vi "Delete Scale.vi"(8 "error in (no error)":errorcluster, 10 "index":i32, 11 "Polynomial Scale configuration in":refnum<class "Polynomial Scale configuration.lvclass">) -> (0 "error out":errorcluster, 3 "Polynomial Scale configuration out":refnum<class "Polynomial Scale configuration.lvclass">)   [LabVIEW 2013, in "Polynomial Scale configuration.lvclass"]
uses:
  Polynomial Scale configuration.lvclass
  <vilib>/NI/DCAF Modules/DCAF Scaling/module/configuration/Scaling configuration.lvclass
  Polynomial Scale configuration.lvclass/Polynomial Scale configuration.ctl
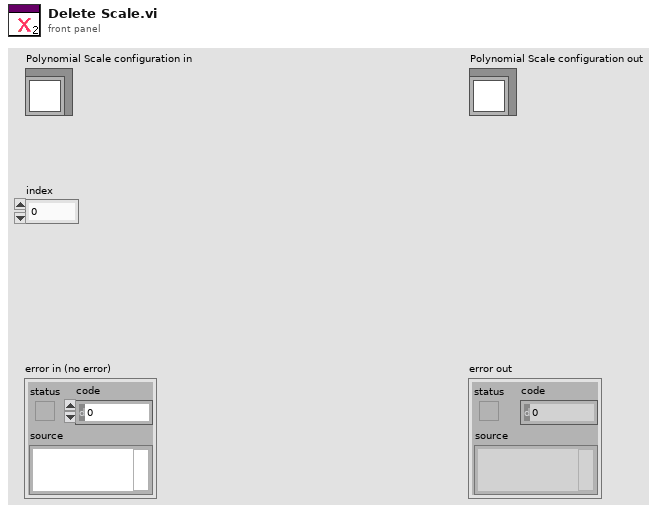
[diagram p1: front panel]
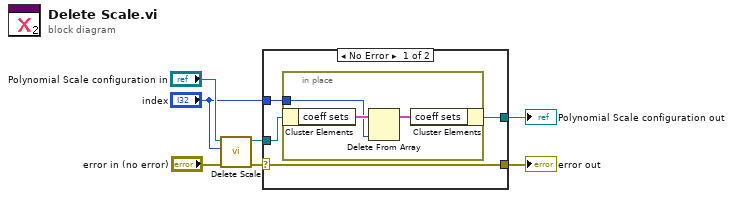
[diagram p0: block diagram]
diagram:
  n1 = call-parent "Delete Scale.vi"("error in (no error)"="error in (no error)", "index"="index", "Scaling configuration in"="Polynomial Scale configuration in") -> ("error out"=w3:errorcluster, "Scaling configuration out"=w1:refnum<class "Polynomial Scale configuration.lvclass">)  [unwired: 7 in]
  n2 = case shown="No Error" w3 {
    selector: w3 -> [w9 w15]
    tunnel: "index" -> [w11 _]
    tunnel: [w10 w16] -> w4
    tunnel: [w9 w15] -> w2
    tunnel: w1 -> [w8 w16]
    frame No Error {
      n3 = in-place {
        in-place-border: w11 -> [w12]
        n4 = in-place-cluster #1(w8) -> ("coeff sets"=w14:cluster{"coeffs":dbl[]}[])
        n5 = Delete From Array(array=w14, index=w12) -> (array with subset deleted=w13:cluster{"coeffs":dbl[]}[])  [unwired: 1 in, 1 out]
        n6 = in-place-cluster #1("coeff sets"=w13) -> (w10:refnum<class "Polynomial Scale configuration.lvclass">)
      }
    }
    frame Error {
    }
  }
  "error out" <- w2
  "Polynomial Scale configuration out" <- w4
